vi "FTW-Actor-SpawnNewInstance.vi"(0 "Instance Configuration":string="{\n  \"Identity\": \"ActorName\",\n  \"InboxAddress\": \"tcp://127.0.0.1:*\",\n  \"HandshakeTimeout\": 1000,\n  \"DebugEnableInboxLogging\": false,\n  \"DebugEnableJobLogging\": false,\n  \"DebugShowPanel\": false\n}", 11 "error in":errorcluster) -> (4 "FTW Actor Connector":refnum<data-value>, 6 "Instance Inbox Address":string, 8 "Instance VI Clone Name":string, 15 "error out":errorcluster)   [LabVIEW 2014]
uses:
  socket/connector/core/FTW-Connector-Core-Type.ctl
  error/FTW-ERR-ThrowError.vi
  error/FTW-ERR-StatusException.vi
  lib/FTW-KernelFilepath.vi
  error/FTW-ERR-CallChain.vi
  string/FTW-STR-ReplaceWhitespace.vi
  json/core/FTW-JSON-Core-EncodingFlags.vi
  reflection/FTW-Reflection-Type.vi
  codegen/xnode/json/fetch/FTW-JSON-Core-GetFlattenedValue.vi
  codegen/xnode/FTW-JSON-Fetch.xnode
panel:
  # "Inputs"
  # "Outputs"
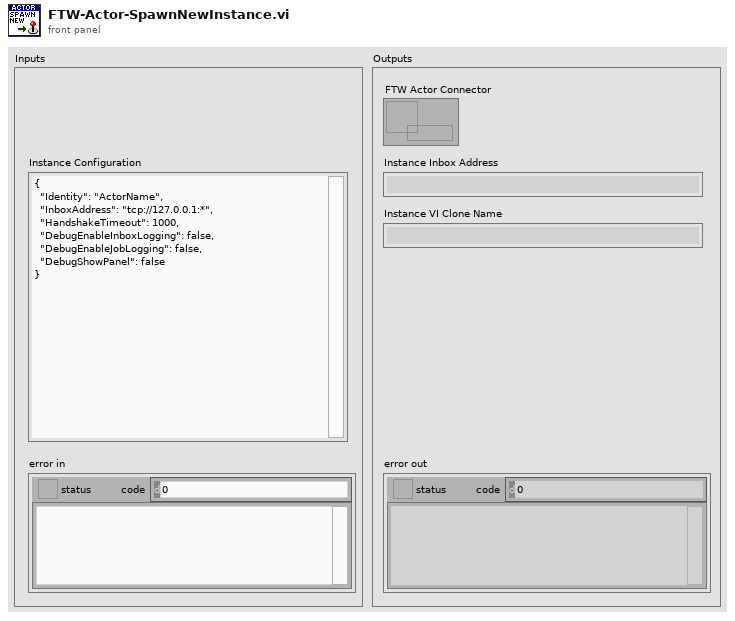
[diagram p1: front panel]
types:
  T1 = cluster{"FTW-PrimaryInboxAddress":string, "FTW-InstanceCloneName":string}
  T2 = cluster{"DebugShowPanel":bool, "ActorInstanceVIFilepath":path, "ActorInstanceVIName":string, "HandshakeTimeout":i32}
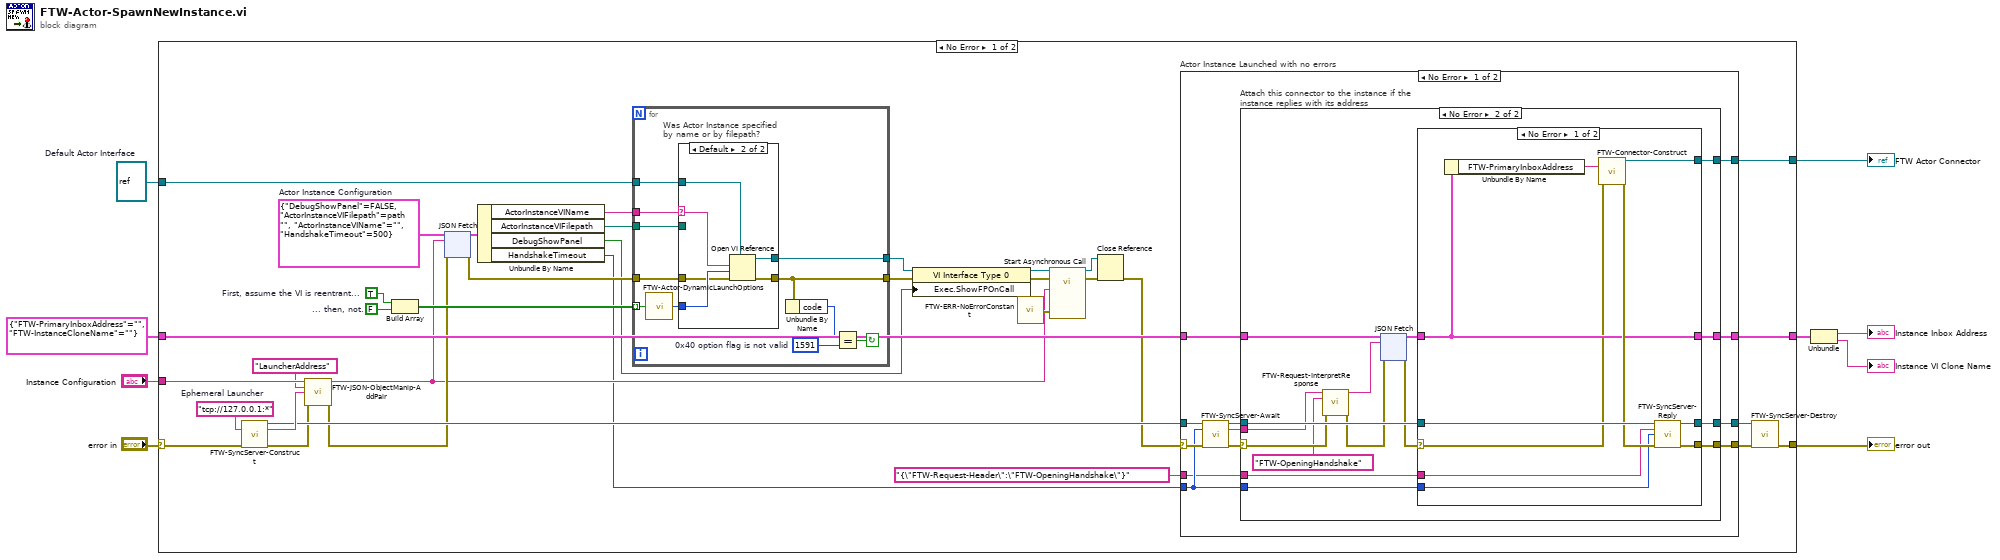
[diagram p0: block diagram]
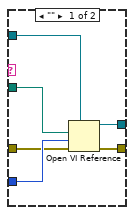
[diagram p2: hidden frame]
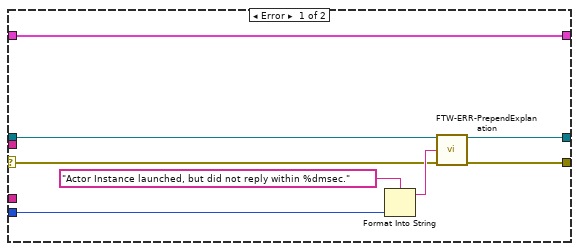
[diagram p3: hidden frame]
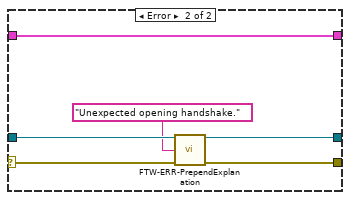
[diagram p4: hidden frame]
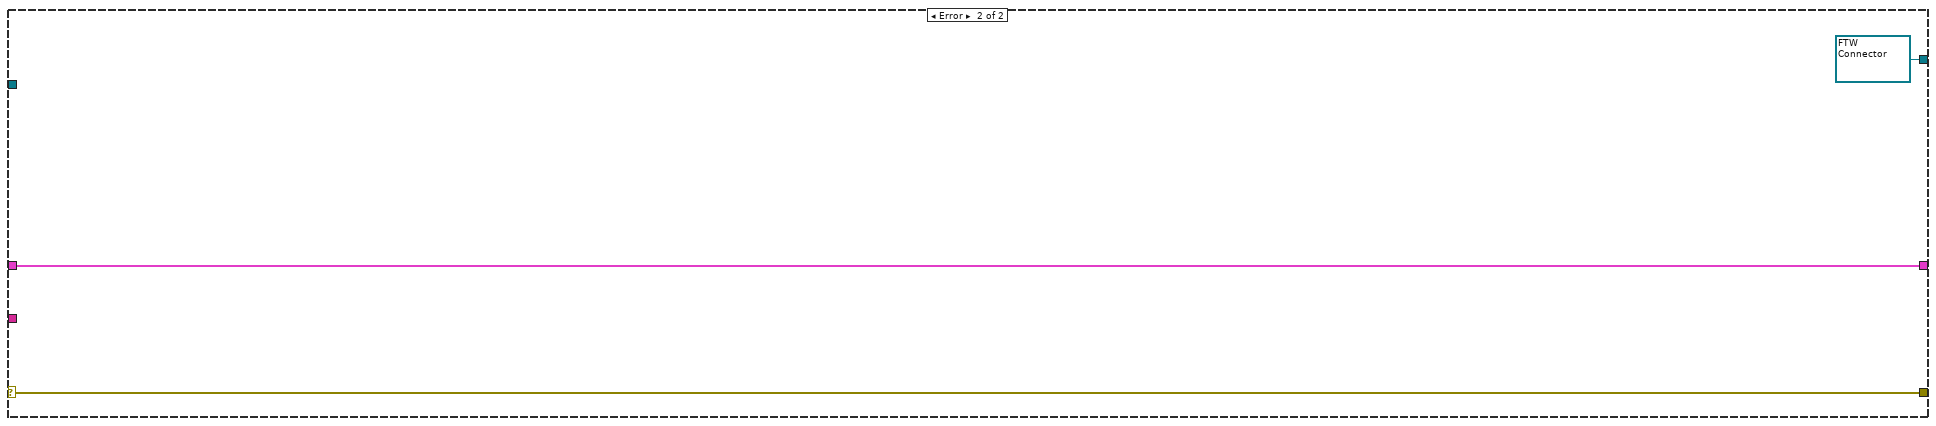
[diagram p6: hidden frame]
diagram:
  w1 = refnum<vi> refnum  # Default Actor Interface
  n1 = case shown="No Error" "error in" {
    selector: "error in" -> [w35 w244]
    tunnel: [w39 w244] -> w6
    tunnel: [w44 refnum<data-value> refnum ("FTW Actor Connector")] -> w7
    tunnel: "Instance Configuration" -> [w43 _]
    tunnel: T1 {"FTW-PrimaryInboxAddress"="", "FTW-InstanceCloneName"=""} -> [w33 w243]
    tunnel: [w32 w243] -> w4
    tunnel: w1 -> [w11 _]
    frame No Error {
      w20 = FALSE  # ... then, not.
      w19 = TRUE  # First, assume the VI is reentrant...
      w29 = T2 {"DebugShowPanel"=FALSE, "ActorInstanceVIFilepath"=path "", "ActorInstanceVIName"="", "HandshakeTimeout"=500}  # Actor Instance Configuration
      w38 = "tcp://127.0.0.1:*"  # Ephemeral Launcher
      n2 = call "FTW-SyncServer-Construct.vi"("Instance Inbox Address"=w38, "error in"=w35) -> ("FTW Synchronous Server"=w36:refnum<data-value>, "Resolved Inbox Address"=w37:string, "error out"=w34:errorcluster)  [unwired: 11 in]
      n3 = call "FTW-JSON-ObjectManip-AddPair.vi"("Input JSON Object"=w43, "Key"="LauncherAddress", "Value"=w37, "error in"=w34) -> ("Output JSON Object"=w14:string, "error out"=w15:errorcluster)  [unwired: 10 in]
      n4 = Build Array(w19, w20) -> (w21:bool[])
      n5 = xnode "JSON Fetch"("Type and Defaults"=w29, "JSON String"=w14, "error in"=w15) -> ("Values"=w31:T2, "error out"=w30:errorcluster)  [unwired: 1 in]
      n6 = Unbundle By Name(w31) -> ("ActorInstanceVIName"=w23:string, "ActorInstanceVIFilepath"=w22:path, "DebugShowPanel"=w16:bool, "HandshakeTimeout"=w13:i32)
      n7 = for {
        tunnel: w11 -> [w116]
        tunnel: [w114] -> w17
        tunnel: [w111] -> w18
        tunnel: w21 -> [w113] mode=indexing
        tunnel: w30 -> [w112]
        tunnel: w22 -> [w108]
        tunnel: w23 -> [w107]
        stop <- w109 continue-if-true
        w106 = 1591  # 0x40 option flag is not valid
        n8 = call "FTW-Actor-DynamicLaunchOptions.vi"("Reentrant?"=w113) -> ("Open VI Ref Options"=w115:i32)
        n9 = case "Was Actor Instance specified\nby name or by filepath?" shown="Default" w107 {
          selector: w107 -> [_ w123]
          tunnel: w116 -> [w122 w128]
          tunnel: w115 -> [w121 w127]
          tunnel: [w120 w126] -> w114
          tunnel: w112 -> [w119 w125]
          tunnel: [w118 w124] -> w111
          tunnel: w108 -> [w117 _]
          frame "" {
            n10 = Open VI Reference(type specifier VI Refnum (for type only)=w122, vi path=w117, options=w121, error in (no error)=w119) -> (vi reference=w120:refnum<vi>, error out=w118:errorcluster)  [unwired: 2 in]
          }
          frame Default {
            n11 = Open VI Reference(type specifier VI Refnum (for type only)=w128, vi path=w123, options=w127, error in (no error)=w125) -> (vi reference=w126:refnum<vi>, error out=w124:errorcluster)  [unwired: 2 in]
          }
        }
        n12 = Unbundle By Name(w111) -> ("code"=w110:i32)
        n13 = Equal?(x=w110, y=w106) -> (x = y?=w109:bool)
      }
      n14 = property class="VI Interface Type 0"(reference=w17, error in=w18, "Exec.ShowFPOnCall"=w16) -> (reference out=w24:refnum<vi>, error out=w26:errorcluster)
      n15 = call "FTW-ERR-NoErrorConstant.vi"() -> ("no error"=w28:errorcluster)
      n16 = call-by-ref "Start Asynchronous Call"(reference=w24, error in=w26, "Actor Instance Configuration"=w14, "ErrorIn"=w28) -> (reference out=w25:refnum<vi>, error out=w27:errorcluster)  [unwired: 13 in, 1 out]
      n17 = Close Reference(reference=w25, error in (no error)=w27) -> (error out=w12:errorcluster)
      n18 = case "Actor Instance Launched with no errors" shown="No Error" w12 {
        selector: w12 -> [w135 w241]
        tunnel: [w140 w241] -> w40
        tunnel: [w139 _] -> w44
        tunnel: w36 -> [w137 w240]
        tunnel: [w138 w240] -> w41
        tunnel: [w130 w239] -> w32
        tunnel: w13 -> [w133 _]
        tunnel: w33 -> [w131 w239]
        tunnel: "{\"FTW-Request-Header\":\"FTW-OpeningHandshake\"}" -> [w129 _]
        frame No Error {
          n19 = call "FTW-SyncServer-Await.vi"("FTW Synchronous Server"=w137, "Receive Timeout"=w133, "error in"=w135) -> ("FTW Synchronous Server out"=w136:refnum<data-value>, "Incoming Request"=w132:string, "error out"=w134:errorcluster)  [unwired: 10 in]
          n20 = case "Attach this connector to the instance if the instance replies with its address" shown="No Error" w134 {
            selector: w134 -> [w142 w156]
            tunnel: [w141 w161] -> w140
            tunnel: [_ w162] -> w139
            tunnel: w136 -> [w147 w158]
            tunnel: [w147 w159] -> w138
            tunnel: w133 -> [w145 w160]
            tunnel: w132 -> [_ w155]
            tunnel: w131 -> [w144 w153]
            tunnel: [w144 w157] -> w130
            tunnel: w129 -> [_ w148]
            frame Error {
              n21 = Format Into String(format string="Actor Instance launched, but did not reply within %dmsec." ("Error Message"), w145) -> (resulting string=w143:string)  [unwired: 2 in, 1 out]
              n22 = call "FTW-ERR-PrependExplanation.vi"("Exception Information"=w143, "error in"=w142) -> ("error out"=w141:errorcluster)  [unwired: 13 in]
            }
            frame No Error {
              n23 = call "FTW-Request-InterpretResponse.vi"("Raw Request"=w155, "Request Header"="FTW-OpeningHandshake", "error in"=w156) -> ("JSON Response"=w149:string, "error out"=w151:errorcluster)  [unwired: 11 in]
              n24 = xnode "JSON Fetch"("Type and Defaults"=w153, "JSON String"=w149, "error in"=w151) -> ("Values"=w152:T1, "error out"=w150:errorcluster)  [unwired: 1 in]
              n25 = case shown="No Error" w150 {
                selector: w150 -> [w227 w235]
                tunnel: [w233 _] -> w162
                tunnel: [w225 w238] -> w161
                tunnel: w152 -> [w229 w236]
                tunnel: w158 -> [w231 w237]
                tunnel: w160 -> [w228 _]
                tunnel: [w226 w237] -> w159
                tunnel: [w229 w236] -> w157
                tunnel: w148 -> [w224 _]
                frame No Error {
                  n26 = Unbundle By Name(w229) -> ("FTW-PrimaryInboxAddress"=w232:string)
                  n27 = call "FTW-Connector-Construct.vi"("Remote Inbox Address"=w232, "error in"=w227) -> ("FTW Actor Connector"=w233:refnum<data-value>, "error out"=w230:errorcluster)  [unwired: 12 in]
                  n28 = call "FTW-SyncServer-Reply.vi"("FTW Synchronous Server"=w231, "Response"=w224, "Send Timeout"=w228, "error in"=w230) -> ("FTW Synchronous Server out"=w226:refnum<data-value>, "error out"=w225:errorcluster)  [unwired: 10 in]
                }
                frame Error {
                  n29 = call "FTW-ERR-PrependExplanation.vi"("Exception Information"="Unexpected opening handshake.", "error in"=w235) -> ("error out"=w238:errorcluster)  [unwired: 13 in]
                }
              }
            }
          }
        }
        frame Error {
        }
      }
      n30 = call "FTW-SyncServer-Destroy.vi"("FTW Synchronous Server"=w41, "error in"=w40) -> ("error out"=w39:errorcluster)  [unwired: 13 in]
    }
    frame Error {
    }
  }
  "error out" <- w6
  "FTW Actor Connector" <- w7
  n31 = Unbundle(w4) -> ("FTW-PrimaryInboxAddress"=→"Instance Inbox Address":string, "FTW-InstanceCloneName"=→"Instance VI Clone Name":string)
